vi "Parse_Origin.vi"(8 "error in (no error)":errorcluster, 11 "JSON String In":string) -> (0 "error out":errorcluster, 1 "Found?":bool, 2 "Origin":string, 3 "JSON String Out":string)   [LabVIEW 2018, in "MerriamWebsterJSON.lvlib"]
uses:
  MerriamWebsterJSON.lvlib
  <vilib>/LVH/i3 JSON/JSON Parsing/Get Array Value at Index Files/Get Array Value at Index - Object.vi
  <vilib>/LVH/i3 JSON/JSON Parsing/Get Object Parameter Files/Get Object Parameter - Object.vi
  <vilib>/LVH/i3 JSON/JSON Parsing/Get Array Value at Index Files/Get Array Value at Index - String.vi
  <vilib>/LVH/i3 JSON/i3-json.lvlib
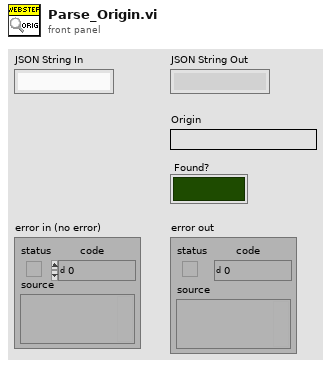
[diagram p1: front panel]
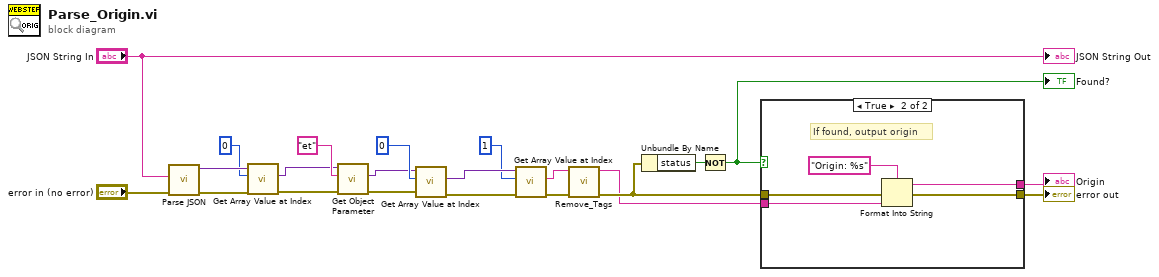
[diagram p0: block diagram]
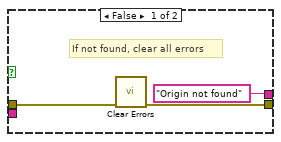
[diagram p2: hidden frame]
diagram:
  n1 = call <vilib>:"Parse JSON.vi"("error in (no error)"="error in (no error)", "JSON String"="JSON String In") -> ("error out"=w20:errorcluster, "JSON Tree"=w21:variant)  [unwired: 6 in, 2 out]
  n2 = call-poly <vilib>:"Get Array Value at Index.vi"("error in (no error)"=w20, "Index"=0, "JSON Tree In (JSON Array)"=w21) -> ("error out"=w16:errorcluster, "JSON Object"=w17:variant)  [unwired: 5 in, 2 out]
  n3 = call-poly <vilib>:"Get Object Parameter.vi"("error in (no error)"=w16, "Parameter Name"="et", "JSON Tree In (JSON Object)"=w17) -> ("error out"=w8:errorcluster, "JSON Object"=w6:variant)  [unwired: 5 in, 2 out]
  n4 = call-poly <vilib>:"Get Array Value at Index.vi"("error in (no error)"=w8, "Index"=0, "JSON Tree In (JSON Array)"=w6) -> ("error out"=w7:errorcluster, "JSON Object"=w12:variant)  [unwired: 5 in, 2 out]
  n5 = call-poly <vilib>:"Get Array Value at Index.vi"("error in (no error)"=w7, "Index"=1, "JSON Tree In (JSON Array)"=w12) -> ("error out"=w3:errorcluster, "String Value"=w4:string)  [unwired: 5 in, 2 out]
  n6 = call "Remove_Tags.vi"("error in (no error)"=w3, "Input String"=w4) -> ("error out"=w2:errorcluster, "Output String"=w1:string)  [unwired: 8 in]
  n7 = Unbundle By Name(w2) -> ("status"=w15:bool)
  n8 = Not(x=w15) -> (.not. x?=w14:bool)
  "Found?" <- w14
  n9 = case shown="True" w14 {
    tunnel: [w25 w30] -> w9
    tunnel: ["Origin not found" ("String Value") w29] -> w13
    tunnel: w2 -> [w23 w28]
    tunnel: w1 -> [_ w27]
    frame False {
      # "If not found, clear all errors"
      n10 = call <vilib>:"Clear Errors.vi"("error in (no error)"=w23) -> ("error out"=w25:errorcluster)  [unwired: 5 in, 1 out]
    }
    frame True {
      # "If found, output origin"
      n11 = Format Into String(format string="Origin: %s", error in=w28, w27) -> (resulting string=w29:string, error out=w30:errorcluster)  [unwired: 1 in]
    }
  }
  "error out" <- w9
  "Origin" <- w13
  "JSON String Out" <- "JSON String In"
